vi "GEN_User Defined Error.vi"() -> (1 "codes":i32[](array[numeric])=[-8001], 2 "descriptions":string[](array[string])=["1111"])   [LabVIEW 2016]
uses:
  <vilib>/Utility/error.llb/DialogType.ctl
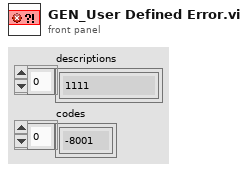
[diagram p1: front panel]
types:
  T1 = typedef "DialogType.ctl" = u16
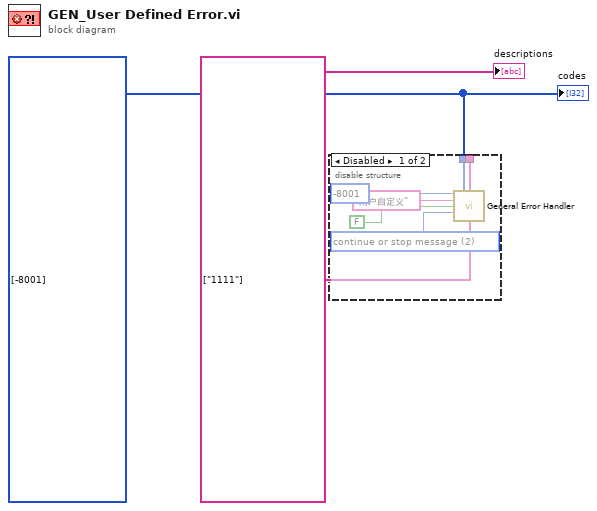
[diagram p0: block diagram]
diagram:
  w1 = string[] ["1111"] ("[user-defined descriptions]")
  w2 = i32[] [-8001] ("[user-defined codes]")
  n1 = disable-structure shown="Disabled" {
    disable-tunnel: w2 -> [w7 _]
    disable-tunnel: w1 -> [w6 _]
    frame Disabled {
      w3 = T1 2 items=["no dialog", "OK message", "continue or stop message", "OK message + warnings", "continue/stop + warnings"] ("type of dialog (OK msg:1)")
      n2 = call <vilib>:"General Error Handler.vi"("[error code] (0)"=-8001 ("error code (no error:0)"), "[user-defined codes]"=w7, "[user-defined descriptions]"=w6, "[error source] (\" \")"="用户自定义" ("[error source] (\" \")"), "search ni.com link visible?(T)"=FALSE, "type of dialog (OK msg:1)"=w3) -> ()  [unwired: 5 in, 5 out]
    }
    frame Enabled {
    }
  }
  "descriptions" <- w1
  "codes" <- w2
